vi "SetEvaluations.vi"(8 "Error In":errorcluster, 9 "Value":string, 10 "Label":string, 11 "reference in":refnum<class "UserManager.lvclass">) -> (0 "Error Out":errorcluster, 3 "reference in":refnum<class "UserManager.lvclass">)   [LabVIEW 2021, in "UserMananger.lvlib" / "UserManager.lvclass"]
uses:
  UserManager.lvclass
  Interface_TAF_AutorizationUpdated/IAuthorizationUpdated/IAuthorizationUpdated.lvclass
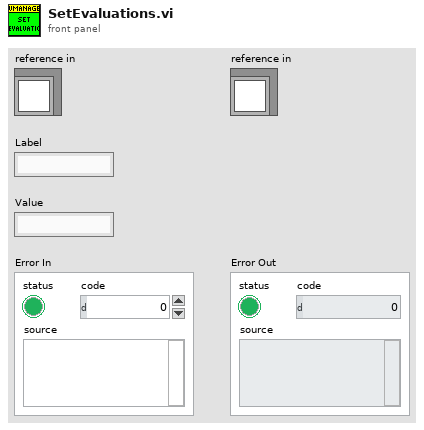
[diagram p1: front panel]
types:
  T1 = typedef "UserMananger.lvlib/UserManager.lvclass/ObjectAttributes.ctl" = cluster{"Interfaces":cluster{"ActivationUpdated":refnum<class "IAuthorizationUpdated.lvclass">}, "Locals":cluster{"MainGUIActive":refnum<queue>, "Evaluations":cluster{"Label":string, "Value":string}[]}, "Persistent":cluster{"Dummy":bool}}
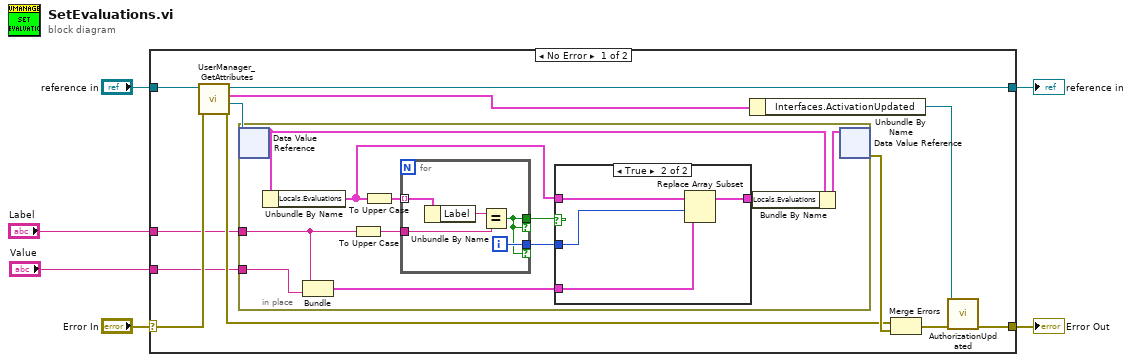
[diagram p0: block diagram]
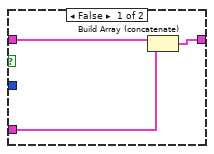
[diagram p2: hidden frame]
diagram:
  n1 = case shown="No Error" "Error In" {
    selector: "Error In" -> [w16 w43]
    tunnel: [w8 w43] -> w5
    tunnel: [w17 w42] -> w3
    tunnel: "reference in" -> [w18 w42]
    tunnel: "Label" -> [w11 _]
    tunnel: "Value" -> [w10 _]
    frame No Error {
      n2 = call "UserManager_GetAttributes.vi"("error in (no error)"=w16, "reference in"=w18) -> ("error out"=w13:errorcluster, "DataRef"=w14:refnum<data-value>, "Data"=w9:T1, "reference out"=w17:refnum<class "UserManager.lvclass">)  [unwired: 6 in]
      n3 = in-place {
        in-place-border: w11 -> [w23]
        in-place-border: w10 -> [w22]
        n4 = in-place-dvr #1(w14) -> (w28:T1)  [unwired: 1 out]
        n5 = Unbundle By Name(w28) -> ("Locals.Evaluations"=w19:cluster{"Label":string, "Value":string}[])
        n6 = Bundle("Label"=w23, "Value"=w22) -> (w21:cluster{"Label":string, "Value":string})  [unwired: 1 in]
        n7 = To Upper Case(1:w23) -> (0:w25:string)
        n8 = To Upper Case(1:w19) -> (0:w26:cluster{"Label":string, "Value":string}[])
        n9 = for {
          tunnel: w26 -> [w34] mode=indexing
          tunnel: w25 -> [w32]
          tunnel: [w30] -> w24 if=w30
          tunnel: [w31] -> w20 if=w30
          i -> [w31]
          n10 = Unbundle By Name(w34) -> ("Label"=w33:string)
          n11 = Equal?(x=w33, y=w32) -> (x = y?=w30:bool)
        }
        n12 = case shown="True" w24 {
          tunnel: w19 -> [w37 w41]
          tunnel: [w36 w40] -> w27
          tunnel: w21 -> [w35 w38]
          tunnel: w20 -> [_ w39]
          frame False {
            n13 = Build Array (concatenate)(w37, w35) -> (w36:cluster{"Label":string, "Value":string}[])
          }
          frame True {
            n14 = Replace Array Subset(array=w41, new element=w38, index=w39) -> (w40:cluster{"Label":string, "Value":string}[])
          }
        }
        n15 = Bundle By Name(cluster=w28, "Locals.Evaluations"=w27) -> (w29:T1)
        n16 = in-place-dvr #1(w29) -> (w15:errorcluster)  [unwired: 1 out]
      }
      n17 = Unbundle By Name(w9) -> ("Interfaces.ActivationUpdated"=w7:refnum<class "IAuthorizationUpdated.lvclass">)
      n18 = Merge Errors(w13, w15) -> (w12:errorcluster)
      n19 = call-dynamic "AuthorizationUpdated.vi"("Error In"=w12, "object in"=w7) -> ("Error Out"=w8:errorcluster)  [unwired: 8 in, 1 out]
    }
    frame Error {
    }
  }
  "Error Out" <- w5
  "reference in" <- w3
